vi "Generate_MAIN_UI_response_event.vi"(8 "error in (no error)":errorcluster, 9 "Frontpanel label (MAIN UI responsive? (F))":string="MAIN UI responsive? (F)", 10 "Responsive? (F)":bool, 11 "System Type":string) -> (0 "error out":errorcluster)   [LabVIEW 2012]
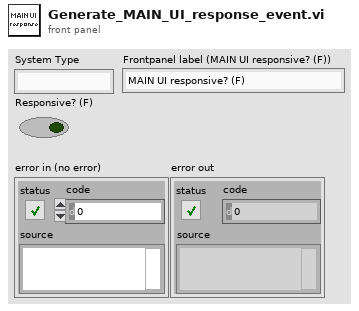
[diagram p1: front panel]
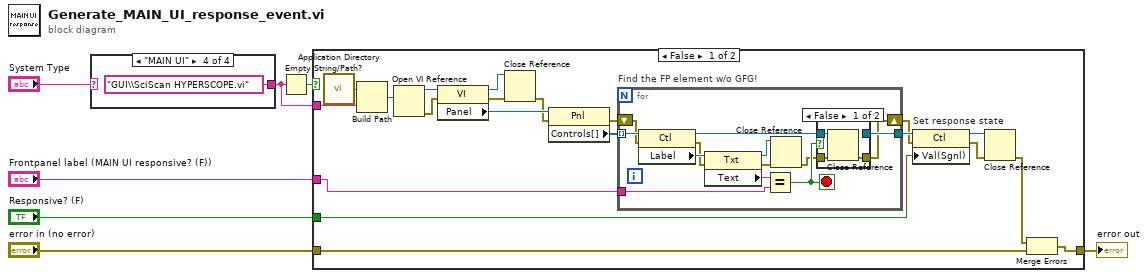
[diagram p0: block diagram]
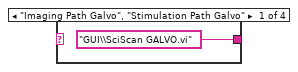
[diagram p4: hidden frame]
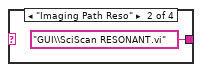
[diagram p5: hidden frame]
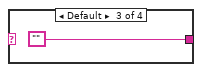
[diagram p6: hidden frame]
diagram:
  n1 = case shown="\"MAIN UI\"" "System Type" {
    tunnel: ["GUI\\SciScan GALVO.vi" ("name or relative path") "GUI\\SciScan RESONANT.vi" ("name or relative path") "" "GUI\\SciScan HYPERSCOPE.vi" ("name or relative path")] -> w5
    frame "Imaging Path Galvo", "Stimulation Path Galvo" {
    }
    frame "Imaging Path Reso" {
    }
    frame Default {
    }
    frame "MAIN UI" {
    }
  }
  n2 = Empty String/Path?(string/path=w5) -> (empty?=w6:bool)
  n3 = case shown="False" w6 {
    tunnel: w5 -> [w23 _]
    tunnel: "Responsive? (F)" -> [w19 _]
    tunnel: "error in (no error)" -> [w15 w50]
    tunnel: [w13 w50] -> w2
    tunnel: "Frontpanel label (MAIN UI responsive? (F))" -> [w12 _]
    frame False {
      n4 = call <vilib>:"Application Directory.vi"() -> ("Application Directory"=w30:path)
      n5 = Build Path(base path=w30, name or relative path=w23) -> (appended path=w31:path)
      n6 = Open VI Reference(vi path=w31) -> (vi reference=w25:refnum<vi>, error out=w24:errorcluster)  [unwired: 5 in]
      n7 = property class="VI"(reference=w25, error in=w24) -> (reference out=w27:refnum<vi>, error out=w28:errorcluster, "Panel"=w29:refnum<vi>)
      n8 = Close Reference(reference=w27, error in (no error)=w28) -> (error out=w18:errorcluster)
      n9 = property class="Pnl"(reference=w29, error in=w18) -> (error out=w17:errorcluster, "Controls[]"=w26:refnum<vi>[])  [unwired: 1 out]
      n10 = for "Find the FP element w/o GFG!" {
        tunnel: w26 -> [w44] mode=indexing
        tunnel: w12 -> [w41]
        tunnel: [w36] -> w22
        shift-right: [w32] -> w16
        shift-left: w17 -> [w35]
        stop <- w37 stop-if-true
        n11 = property class="Ctl"(reference=w44, error in=w35) -> (reference out=w38:refnum<vi>, error out=w34:errorcluster, "Label"=w43:refnum<vi>)
        n12 = property class="Txt"(reference=w43, error in=w34) -> (reference out=w40:refnum<vi>, error out=w39:errorcluster, "Text"=w42:string)
        n13 = Equal?(x=w42, y=w41) -> (x = y?=w37:bool)
        n14 = Close Reference(reference=w40, error in (no error)=w39) -> (error out=w33:errorcluster)
        n15 = case shown="False" w37 {
          tunnel: w38 -> [w47 w49]
          tunnel: [_ w49] -> w36
          tunnel: w33 -> [w46 w48]
          tunnel: [w45 w48] -> w32
          frame False {
            n16 = Close Reference(reference=w47, error in (no error)=w46) -> (error out=w45:errorcluster)
          }
          frame True {
          }
        }
      }
      n17 = property on="Set response state" class="Ctl"(reference=w22, error in=w16, "Val(Sgnl)"=w19) -> (reference out=w21:refnum<vi>, error out=w20:errorcluster)
      n18 = Close Reference(reference=w21, error in (no error)=w20) -> (error out=w14:errorcluster)
      n19 = Merge Errors(w14, w15) -> (w13:errorcluster)
    }
    frame True {
    }
  }
  "error out" <- w2
